vi "DSF.Shared.Configuration.Cycle Timed.Get Priority.vi"(8 "error in (no error)":errorcluster, 11 "Cycle Timed Configuration in":refnum<class "DSF.Shared.Configuration.Cycle Timed.lvclass">) -> (0 "error out":errorcluster, 2 "Priority":u8, 3 "Cycle Timed Configuration out":refnum<class "DSF.Shared.Configuration.Cycle Timed.lvclass">)   [LabVIEW 2016, in "DSF.Shared.lvlib" / "DSF.Shared.Configuration.Cycle Timed.lvclass"]
uses:
  DSF.Shared.Configuration.Cycle Timed.lvclass
  DSF.Shared.Configuration.Cycle Timed.lvclass/DSF.Shared.Configuration.Cycle Timed.ctl
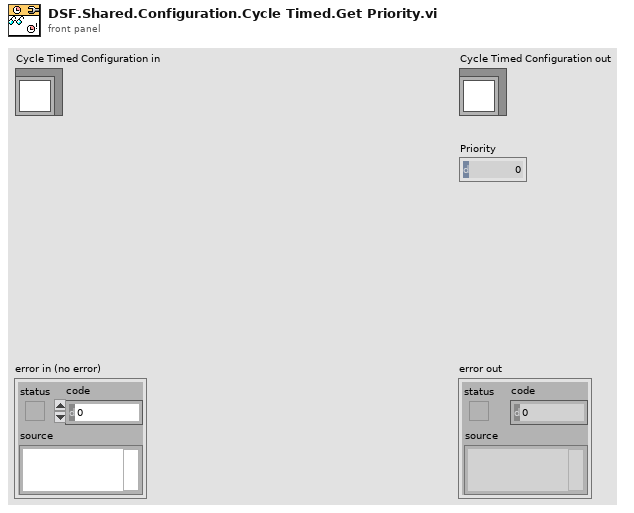
[diagram p1: front panel]
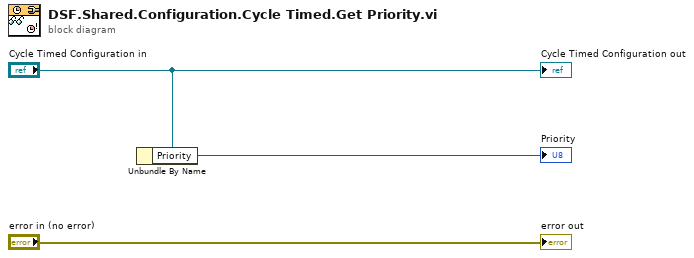
[diagram p0: block diagram]
diagram:
  n1 = Unbundle By Name("Cycle Timed Configuration in") -> ("Priority"=→"Priority":u8)
  "error out" <- "error in (no error)"
  "Cycle Timed Configuration out" <- "Cycle Timed Configuration in"
